vi "Experimental Triangle Half Ramp.vi"(1 "Phase Offset":dbl format="%#_13g") -> (0 "Half Triangle":waveform(dbl))   [LabVIEW 2013]
uses:
  <vilib>/measure/NI_MABase.lvlib
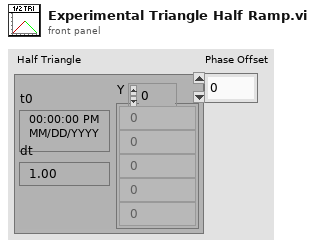
[diagram p1: front panel]
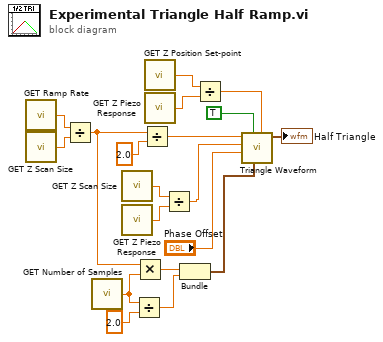
[diagram p0: block diagram]
diagram:
  n1 = call "GET Ramp Rate.vi"() -> ("Ramp Rate"=w3:dbl)
  n2 = call "GET Z Scan Size.vi"() -> ("Z Scan Size"=w2:dbl)
  n3 = Divide(x=w3, y=w2) -> (x/y=w1:dbl)
  n4 = call "GET Number of Samples.vi"() -> ("Number of Samples"=w4:dbl)
  n5 = call "GET Z Scan Size.vi"() -> ("Z Scan Size"=w15:dbl)
  n6 = call "GET Z Piezo Response.vi"() -> ("Z Piezo Response"=w14:dbl)
  n7 = Divide(x=w4, y=2.0) -> (x/y=w6:dbl)
  n8 = Multiply(x=w1, y=w4) -> (x*y=w11:dbl)
  n9 = Divide(x=w1, y=2.0) -> (x/y=w8:dbl)
  n10 = call "GET Z Position Set-point.vi"() -> ("Z Position Set-point"=w17:dbl)
  n11 = call "GET Z Piezo Response.vi"() -> ("Z Piezo Response"=w18:dbl)
  n12 = Divide(x=w15, y=w14) -> (x/y=w13:dbl)
  n13 = Bundle(w11, w6) -> (w12:cluster{dbl, dbl})  [unwired: 1 in]
  n14 = Divide(x=w17, y=w18) -> (x/y=w16:dbl)
  n15 = call <vilib>:"Triangle Waveform.vi"("offset"=w16, "sampling info"=w12, "reset signal"=TRUE, "phase"="Phase Offset", "amplitude"=w13, "frequency"=w8) -> ("signal out"=→"Half Triangle":waveform(dbl))  [unwired: 4 in, 1 out]
